vi "Get Selected Item.vi"(8 "error in (no error)":errorcluster, 11 "Listbox in":refnum<class "Listbox.lvclass">) -> (0 "error out":errorcluster, 2 "Item":refnum<class "Item.lvclass">, 3 "Listbox out":refnum<class "Listbox.lvclass">)   [LabVIEW 2016, in "斯坦道氨氮.lvlib" / "Listbox.lvclass"]
uses:
  Listbox.lvclass
  Interfaces/Item/Item.lvclass
  Listbox.lvclass/Listbox.ctl
panel:
  # "NOTICE -- YOU MUST LEAVE THIS NOTICE IN PLACE.\n\nCopyright (c) 2017, LIANG LIU Shawn.Liu.cn@gmail.com\nAll rights reserved.\n\nRedistribution and use in source and binary forms, with or without modification, are permitted provided that the following conditions are met:\n-Redistributions of source code must retain the above copyright notice, this list of conditions and the following disclaimer.\n-Redistributions in binary form must reproduce the above copyright notice, this list of conditions and the following disclaimer in the documentation and/or other materials provided with the distribution.\n-Neither the name of the eLp nor the names of its contributors may be used to endorse or promote products derived from this software without specific prior written permission.\n\nTHIS SOFTWARE IS PROVIDED BY THE COPYRIGHT HOLDERS AND CONTRIBUTORS \"AS IS\" AND ANY EXPRESS OR IMPLIED WARRANTIES, INCLUDING, BUT NOT LIMITED TO, THE IMPLIED WARRANTIES OF MERCHANTABILITY AND FITNESS FOR A PARTICULAR PURPOSE ARE DISCLAIMED. IN NO EVENT SHALL THE COPYRIGHT HOLDER OR CONTRIBUTORS BE LIABLE FOR ANY DIRECT, INDIRECT, INCIDENTAL, SPECIAL, EXEMPLARY, OR CONSEQUENTIAL DAMAGES (INCLUDING, BUT NOT LIMITED TO, PROCUREMENT OF SUBSTITUTE GOODS OR SERVICES; LOSS OF USE, DATA, OR PROFITS; OR BUSINESS INTERRUPTION) HOWEVER CAUSED AND ON ANY THEORY OF LIABILITY, WHETHER IN CONTRACT, STRICT LIABILITY, OR TORT (INCLUDING NEGLIGENCE OR OTHERWISE) ARISING IN ANY WAY OUT OF THE USE OF THIS SOFTWARE, EVEN IF ADVISED OF THE POSSIBILITY OF SUCH DAMAGE."
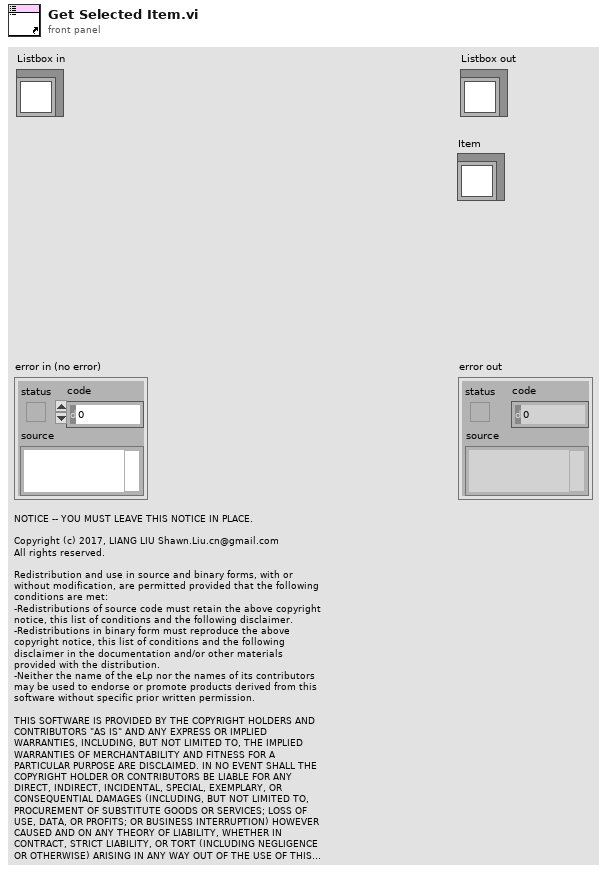
[diagram p1: front panel]
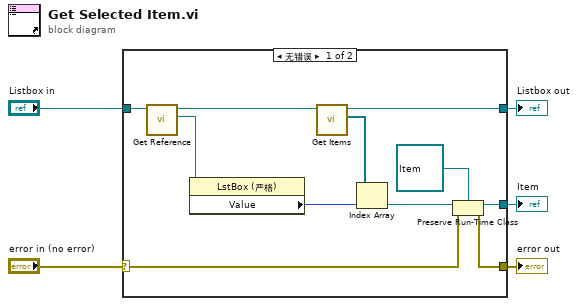
[diagram p0: block diagram]
diagram:
  n1 = case shown="无错误" "error in (no error)" {
    selector: "error in (no error)" -> [w7 w18]
    tunnel: "Listbox in" -> [w16 w17]
    tunnel: [w13 w17] -> w4
    tunnel: [w8 w18] -> w3
    tunnel: [w6 _] -> w1
    frame No Error {
      n2 = call "Get Reference.vi"("Listbox in"=w16) -> ("Reference"=w14:refnum<vi>, "Listbox out"=w15:refnum<class "Listbox.lvclass">)  [unwired: 9 in]
      n3 = property class="LstBox (严格)"(reference=w14) -> ("Value"=w11:i32)  [unwired: 1 in, 2 out]
      n4 = call "Get Items.vi"("Listbox in"=w15) -> ("Items"=w12:refnum<class "Listbox Item.lvclass">[], "Listbox out"=w13:refnum<class "Listbox.lvclass">)  [unwired: 9 in]
      n5 = Index Array(array=w12, index=w11) -> (element=w10:refnum<class "Listbox Item.lvclass">)
      n6 = Preserve Run-Time Class(object in=w10, error in=w7, 2:refnum<class "Item.lvclass"> refnum ("Item.lvclass")) -> (object out=w6:refnum<class "Item.lvclass">, error out=w8:errorcluster)
    }
    frame Error {
    }
  }
  "error out" <- w3
  "Listbox out" <- w4
  "Item" <- w1
